vi "Read Multiple Line Keys.vi"(8 "error in (no error)":errorcluster) -> (0 "error out":errorcluster, 3 "output cluster":T1)   [LabVIEW 2017, in "csm-ini-variable-addon.lvclass"]
uses:
  csm-ini-variable-addon.lvclass
  INI-Static-Variable-Support/LabVIEW-Config/LabVIEW-Config.lvclass
  INI-Static-Variable-Support/LabVIEW-Config/Read Key (Raw).vi
  INI-Static-Variable-Support/LabVIEW-Config/Read Key (Boolean).vi
  INI-Static-Variable-Support/LabVIEW-Config/Read Key (DBL).vi
  INI-Static-Variable-Support/LabVIEW-Config/Read Key (U32).vi
  INI-Static-Variable-Support/LabVIEW-Config/Read Key (I32).vi
panel:
  out "text":string
  out "Config":T2
  out "Value":string
  out "Key Names":string[](array[string])
  out "Section Names":string[](array[string])
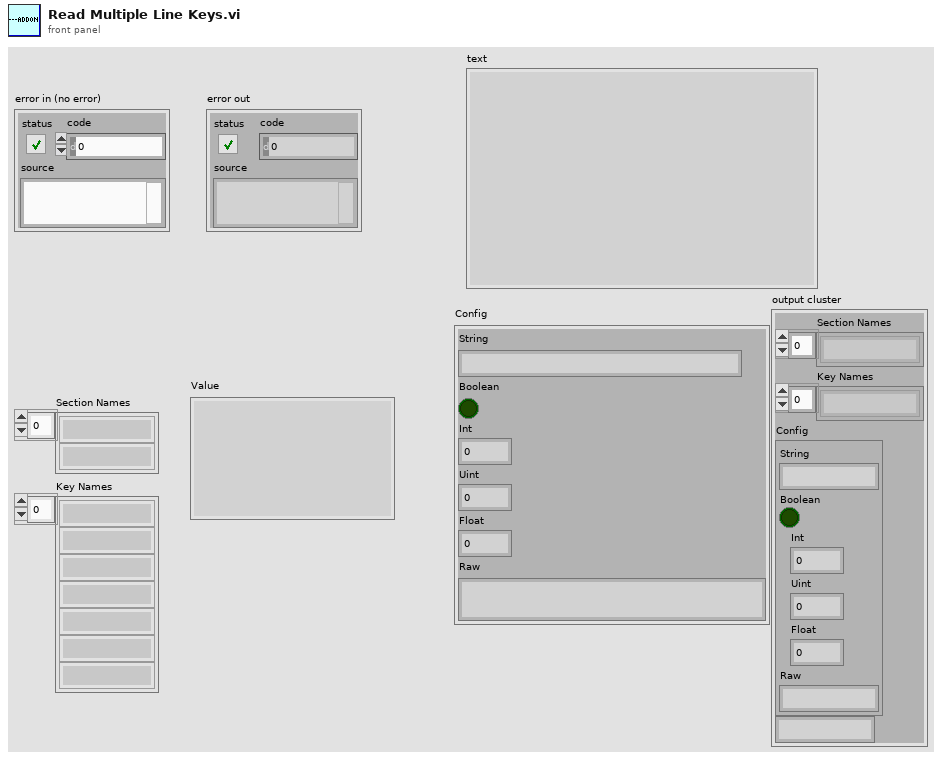
[diagram p1: front panel]
types:
  T1 = cluster{"Section Names":string[], "Key Names":string[], "Config":cluster{"String":string, "Boolean":bool, "Int":i32, "Uint":u32, "Float":dbl, "Raw":string}, string}
  T2 = cluster{"String":string, "Boolean":bool, "Int":i32, "Uint":u32, "Float":dbl, "Raw":string}
  T3 = typedef "LabVIEW-Config.lvlib/LabVIEW-Config.lvclass/Config.ctl" = cluster{"Path":path, "Lines":string[], "Tokens":T4[], "Modified?":bool, "Cache":cluster{"Valid?":bool, "Key Information":T5[]}}
  T4 = typedef "LabVIEW-Config.lvlib/LabVIEW-Config.lvclass/LineToken.ctl" = enum8{"comment", "section", "key", "more"}
  T5 = typedef "LabVIEW-Config.lvlib/LabVIEW-Config.lvclass/KeyInfo.ctl" = cluster{"Key Indexes":cluster{"Indexes":i32[]}[], "Session Found?":bool, "Key found?":bool, "Session Index":i32}
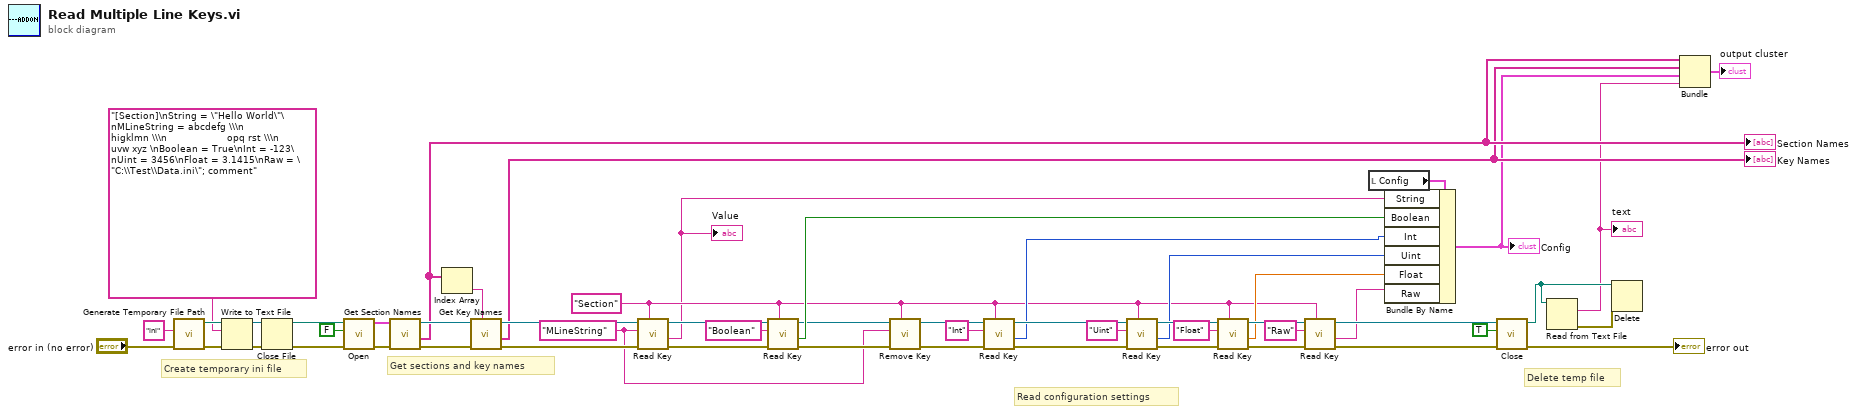
[diagram p0: block diagram]
diagram:
  w10 = "Section" ("Section Name")
  w6 = "MLineString" ("Key Name")
  # "Get sections and key names"
  # "Delete temp file"
  # "Read configuration settings"
  # "Create temporary ini file"
  n1 = call <vilib>:"Generate Temporary File Path.vi"("error in (no error)"="error in (no error)", "Temporary File Extension (tmp)"="ini") -> ("error out"=w45:errorcluster, "Unique Temporary File Path"=w42:path)  [unwired: 8 in]
  n2 = Write to Text File(file (use dialog)=w42, text="[Section]\nString = \"Hello World\"\nMLineString = abcdefg \\\n                    higklmn \\\n                    opq rst \\\n                    uvw xyz \nBoolean = True\nInt = -123\nUint = 3456\nFloat = 3.1415\nRaw = \"C:\\Test\\Data.ini\"; comment", error in=w45) -> (refnum out=w41:refnum<file>, error out=w43:errorcluster)  [unwired: 1 in, 1 out]
  n3 = Close File(refnum=w41, error in=w43) -> (path=w27:path, error out=w28:errorcluster)
  n4 = call "Open.vi"("error in (no error)"=w28, "Create if not exists? (T)"=FALSE, "Path"=w27) -> ("error out"=w52:errorcluster, "Config"=w25:T3)  [unwired: 5 in, 2 out]
  n5 = call "Get Section Names.vi"("error in (no error)"=w52, "Config in"=w25) -> ("error out"=w26:errorcluster, "Section Names"=w5:string[], "Config out"=w23:refnum<class "LabVIEW-Config.lvclass">)  [unwired: 7 in]
  "Section Names" <- w5
  n6 = Index Array(array=w5) -> (element=w21:string)  [unwired: 1 in]
  n7 = call "Get Key Names.vi"("Section Name"=w21, "error in (no error)"=w26, "Config in"=w23) -> ("error out"=w24:errorcluster, "Key Names"=w4:string[], "Config out"=w22:refnum<class "LabVIEW-Config.lvclass">)  [unwired: 5 in, 1 out]
  "Key Names" <- w4
  n8 = call-poly "Read Key.vi"("Section Name"=w10, "error in (no error)"=w24, "Key Name"=w6, "Config in"=w22) -> ("error out"=w50:errorcluster, "Content"=w9:string, "Config out"=w49:refnum<class "LabVIEW-Config.lvclass">)  [unwired: 4 in, 1 out]
  "Value" <- w9
  n9 = call-poly "Read Key.vi"("Section Name"=w10, "error in (no error)"=w50, "Key Name"="Boolean", "Config in"=w49) -> ("error out"=w12:errorcluster, "Value"=w19:bool, "Config out"=w13:refnum<class "LabVIEW-Config.lvclass">)  [unwired: 4 in, 1 out]
  n10 = call "Remove Key.vi"("Section Name"=w10, "error in (no error)"=w12, "Key Name"=w6, "Config in"=w13) -> ("error out"=w11:errorcluster, "Config out"=w14:refnum<class "LabVIEW-Config.lvclass">)  [unwired: 5 in, 1 out]
  n11 = call-poly "Read Key.vi"("Section Name"=w10, "error in (no error)"=w11, "Key Name"="Int", "Config in"=w14) -> ("error out"=w48:errorcluster, "Value"=w18:i32, "Config out"=w39:refnum<class "LabVIEW-Config.lvclass">)  [unwired: 4 in, 1 out]
  n12 = call-poly "Read Key.vi"("Section Name"=w10, "error in (no error)"=w48, "Key Name"="Uint", "Config in"=w39) -> ("error out"=w40:errorcluster, "Value"=w17:u32, "Config out"=w36:refnum<class "LabVIEW-Config.lvclass">)  [unwired: 4 in, 1 out]
  n13 = call-poly "Read Key.vi"("Section Name"=w10, "error in (no error)"=w40, "Key Name"="Float", "Config in"=w36) -> ("error out"=w37:errorcluster, "Value"=w16:dbl, "Config out"=w32:refnum<class "LabVIEW-Config.lvclass">)  [unwired: 4 in, 1 out]
  n14 = call-poly "Read Key.vi"("Section Name"=w10, "error in (no error)"=w37, "Key Name"="Raw", "Config in"=w32) -> ("error out"=w33:errorcluster, "Content"=w15:string, "Config out"=w31:refnum<class "LabVIEW-Config.lvclass">)  [unwired: 4 in, 1 out]
  n15 = local read "Config"() -> (w20:T2)
  n16 = Bundle By Name(cluster=w20, "String"=w9, "Boolean"=w19, "Int"=w18, "Uint"=w17, "Float"=w16, "Raw"=w15) -> (w3:T2)
  "Config" <- w3
  n17 = call "Close.vi"("error in (no error)"=w33, "Write if modified? (T)"=TRUE, "Config"=w31) -> ("error out"=→"error out":errorcluster, "Path"=w8:path)  [unwired: 7 in]
  n18 = Read from Text File(file (use dialog)=w8) -> (text=w2:string, error out=w7:errorcluster)  [unwired: 3 in, 2 out]
  "text" <- w2
  n19 = Delete(path (use dialog)=w8, error in=w7) -> ()  [unwired: 3 in, 3 out]
  n20 = Bundle("Section Names"=w5, "Key Names"=w4, "Config"=w3, w2) -> (→"output cluster":T1)  [unwired: 1 in]
